vi "CreateTagsFromItemNames.vi"(8 "error in":errorcluster, 10 "item names":string[](array[string]), 11 "item tags":string[](array[string])) -> (0 "error out":errorcluster, 2 "item names":string[](array[string]), 3 "item tags":string[](array[string]))   [LabVIEW 2021, in "Menu.lvlib" / "Menu.lvclass"]
uses:
  Menu.lvclass
  <vilib>/Utility/error.llb/Error Cluster From Error Code.vi
  <vilib>/ErrorRing/Error Ring.xnode
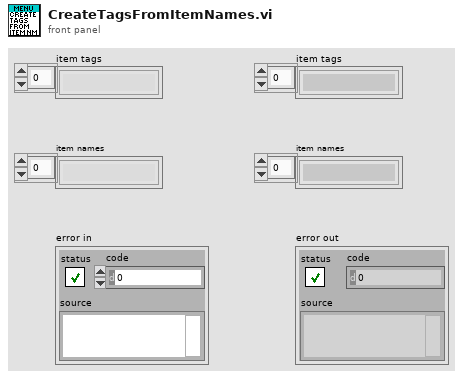
[diagram p1: front panel]
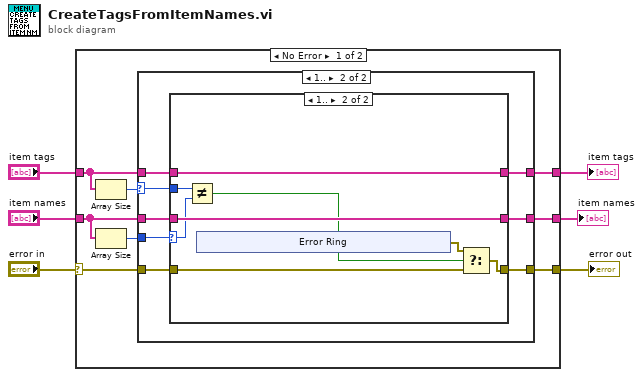
[diagram p0: block diagram]
diagram:
  n1 = case shown="No Error" "error in" {
    selector: "error in" -> [w10 w51]
    tunnel: [w9 w51] -> w6
    tunnel: "item tags" -> [w11 w50]
    tunnel: [w14 w50] -> w4
    tunnel: "item names" -> [w12 w49]
    tunnel: [w13 w49] -> w3
    frame No Error {
      n2 = Array Size(array=w11) -> (size(s)=w8:i32)
      n3 = Array Size(array=w12) -> (size(s)=w7:i32)
      n4 = case shown="1.." w8 {
        selector: w8 -> [_ w27]
        tunnel: [w19 w34] -> w14
        tunnel: w7 -> [w21 w33]
        tunnel: [w17 w32] -> w13
        tunnel: w12 -> [w18 w31]
        tunnel: w11 -> [w20 w30]
        tunnel: w10 -> [w16 w29]
        tunnel: [w15 w28] -> w9
        frame ..0 {
          n5 = case shown="..0" w21 {
            tunnel: [w24 w26] -> w19
            tunnel: w20 -> [w24 _]
            tunnel: [w23 w26] -> w17
            tunnel: w18 -> [w23 w26]
            tunnel: [w22 w25] -> w15
            tunnel: w16 -> [w22 w25]
            frame ..0 {
            }
            frame 1.. {
            }
          }
        }
        frame 1.. {
          n6 = case shown="1.." w33 {
            selector: w33 -> [_ w37]
            tunnel: w30 -> [w35 w44]
            tunnel: [w35 w44] -> w34
            tunnel: w31 -> [_ w43]
            tunnel: [w35 w43] -> w32
            tunnel: w29 -> [w36 w42]
            tunnel: [w36 w41] -> w28
            tunnel: w27 -> [_ w38]
            frame ..0 {
            }
            frame 1.. {
              n7 = Not Equal?(x=w38, y=w37) -> (x != y?=w40:bool)
              n8 = xnode "Error Ring"() -> ("error out"=w39:errorcluster)
              n9 = Select(t=w39, s=w40, f=w42) -> (s? t:f=w41:errorcluster)
            }
          }
        }
      }
    }
    frame Error {
    }
  }
  "item names" <- w3
  "item tags" <- w4
  "error out" <- w6
